vi "PAS_CmdStr_390.vi"(1 "PAS命令输入":T1 {"倒车雷达右后区距离" items=["无距离", "Range1", "Range2", "Range3", "Range4", "Range5", "Range6", "Range7"]; "倒车雷达右后中区距离" items=["无距离", "Range1", "Range2", "Range3", "Range4", "Range5", "Range6", "Range7"]; "倒车雷达左后中区距离" items=["无距离", "Range1", "Range2", "Range3", "Range4", "Range5", "Range6", "Range7"]; "倒车雷达左后区距离" items=["无距离", "Range1", "Range2", "Range3", "Range4", "Range5", "Range6", "Range7"]; "倒车雷达右前区距离" items=["无距离", "Range1", "Range2", "Range3", "Range4", "Range5", "Range6", "Range7"]; "倒车雷达右中前区距离" items=["无距离", "Range1", "Range2", "Range3", "Range4", "Range5", "Range6", "Range7"]; "倒车雷达左中前区距离" items=["无距离", "Range1", "Range2", "Range3", "Range4", "Range5", "Range6", "Range7"]; "倒车雷达左前区距离" items=["无距离", "Range1", "Range2", "Range3", "Range4", "Range5", "Range6", "Range7"]; "倒车雷达工作方式" items=["关闭", "待机", "前后激活", "前激活", "后激活", "系统错误", "禁止", "无效"]; "蜂鸣器报警方式" items=["关闭", "前蜂鸣开", "前蜂鸣4Hz", "前蜂鸣2Hz", "后蜂鸣开", "后蜂鸣4Hz", "后蜂鸣2Hz", "预留"]}) -> (0 "CmdStr":string)   [LabVIEW 2013]
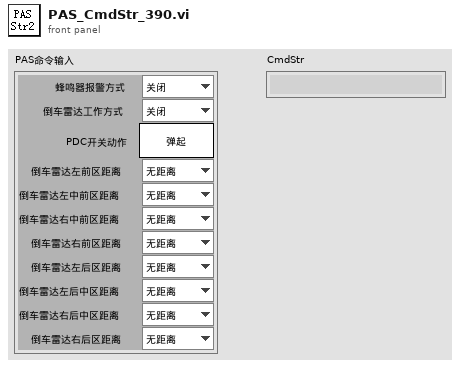
[diagram p1: front panel]
types:
  T1 = cluster{"蜂鸣器报警方式":u8, "倒车雷达工作方式":u8, "PDC开关动作":bool, "倒车雷达左前区距离":u8, "倒车雷达左中前区距离":u8, "倒车雷达右中前区距离":u8, "倒车雷达右前区距离":u8, "倒车雷达左后区距离":u8, "倒车雷达左后中区距离":u8, "倒车雷达右后中区距离":u8, "倒车雷达右后区距离":u8}
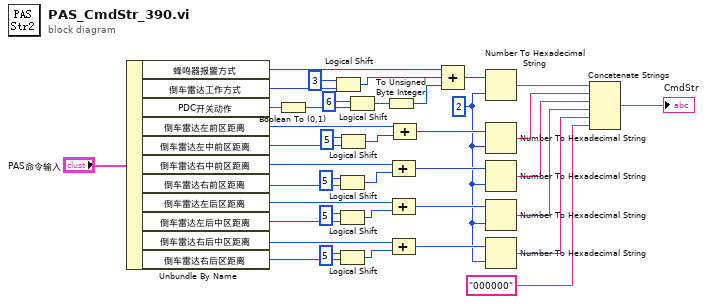
[diagram p0: block diagram]
diagram:
  w7 = 2
  n1 = Unbundle By Name("PAS命令输入") -> ("蜂鸣器报警方式"=w38:u8, "倒车雷达工作方式"=w36:u8, "PDC开关动作"=w34:bool, "倒车雷达左前区距离"=w27:u8, "倒车雷达左中前区距离"=w28:u8, "倒车雷达右中前区距离"=w21:u8, "倒车雷达右前区距离"=w20:u8, "倒车雷达左后区距离"=w19:u8, "倒车雷达左后中区距离"=w18:u8, "倒车雷达右后中区距离"=w15:u8, "倒车雷达右后区距离"=w14:u8)
  n2 = Boolean To (0,1)(Boolean=w34) -> (0, 1=w32:i16)
  n3 = Logical Shift(y=u8 3, x=w36) -> (x << y=w35:u8)
  n4 = Logical Shift(y=u8 5, x=w20) -> (x << y=w25:u8)
  n5 = Logical Shift(y=u8 5, x=w18) -> (x << y=w22:u8)
  n6 = Logical Shift(y=u8 5, x=w14) -> (x << y=w17:u8)
  n7 = Logical Shift(y=u8 5, x=w28) -> (x << y=w26:u8)
  n8 = Logical Shift(y=u8 6, x=w32) -> (x << y=w31:i16)
  n9 = To Unsigned Byte Integer(number=w31) -> (unsigned 8bit integer=w30:u8)
  n10 = Compound Arithmetic op=ADD(w21, w25) -> (w10:u8)
  n11 = Compound Arithmetic op=ADD(w19, w22) -> (w9:u8)
  n12 = Compound Arithmetic op=ADD(w15, w17) -> (w8:u8)
  n13 = Compound Arithmetic op=ADD(w27, w26) -> (w11:u8)
  n14 = Compound Arithmetic op=ADD(w38, w35, w30) -> (w13:u8)
  n15 = Number To Hexadecimal String(1:w7, 2:w13) -> (0:w12:string)
  n16 = Number To Hexadecimal String(1:w7, 2:w11) -> (0:w6:string)
  n17 = Number To Hexadecimal String(1:w7, 2:w10) -> (0:w5:string)
  n18 = Number To Hexadecimal String(1:w7, 2:w9) -> (0:w4:string)
  n19 = Number To Hexadecimal String(1:w7, 2:w8) -> (0:w3:string)
  n20 = Concatenate Strings(w12, w6, w5, w4, w3, "000000") -> (→"CmdStr":string)
